vi "ProcessInfoGui.vi"() -> (1 "cancel":bool, 2 "PlateType":T1)   [LabVIEW 2016]
uses:
  Sequence/Sequence.PlateType.ctl
  InfoGui.Action.ctl
  tools/Translator/Translator.Message.ctl
  tools/Translator/Translator.FormatMessage.vi
  Sequence/Sequence.Global.vi
  Global/ApplicationGlobal.vi
  tools/Translator/Translator.Global.vi
panel:
  in  "CancelButton":bool
  in  "ClientPlateSelect":bool
  in  "WabcoPlateSelect":bool
  out "Message":string
  out "Client Plate Status":string caption="Status tabliczki Klienta"
  out "ClientPlate":picture
  out "Wabco Plate Status":string caption="Status tabliczki Wabco"
  out "WabcoPlate":picture
  out "_loop":i32(ring)=4
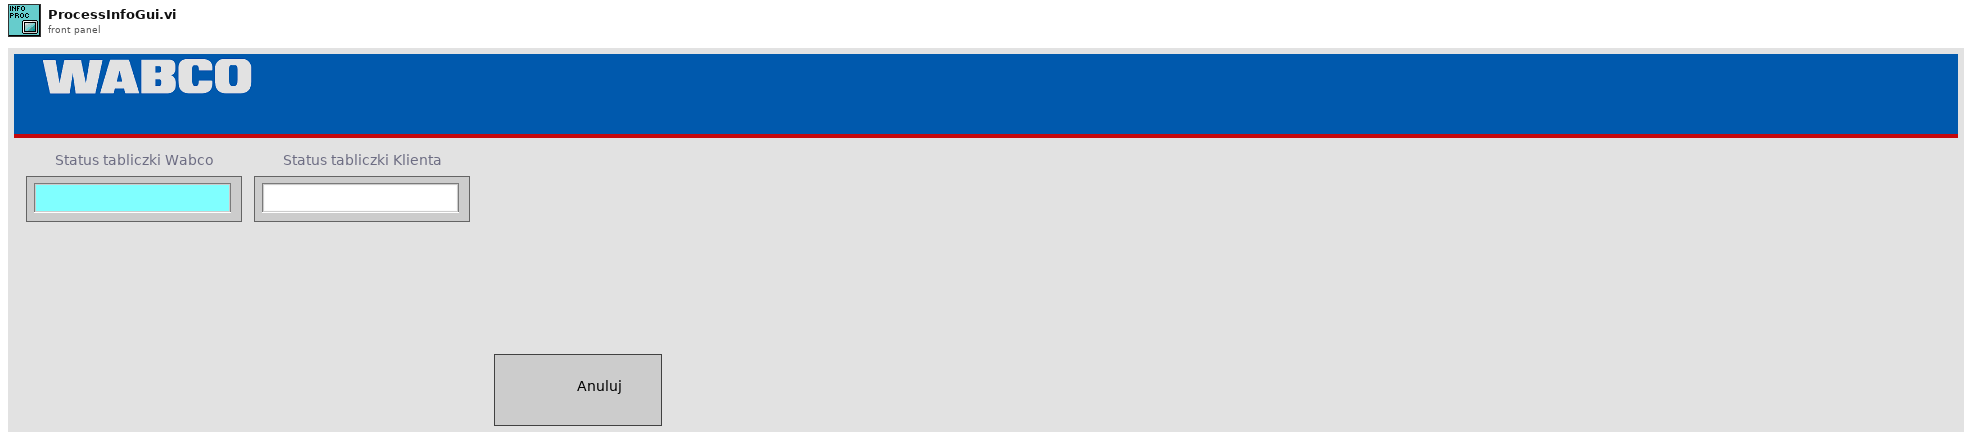
[diagram p1: front panel]
types:
  T1 = typedef "Sequence.PlateType.ctl" = enum16{"Wabco", "Client"}
  T2 = typedef "InfoGui.Action.ctl" = enum32{"idle", "constructor", "destructor", "--- InfoGUI ---"}
  T3 = typedef "Translator.Message.ctl" = enum16{"-", "Event confirmed", "Log out", "Log in", "Shutdown", "Cancel", "Start", "Begin time", "End time", "Duration", "Service Mode", "Ignore Results", "Serial Format", "On", "Off", "OK", "NOK", "NOK %s", "Home", "Work", "Close", "Open", "In progress...", "Missing", "Empty", "Hardware failure", "Initial", "Default", "Total", "Out of range", "Free disk space is below 1GB - contact technician", "Error %d >> %s", "Error %d >> %s >> %s", "Msg %d >> %s", "Laser msg %d %s", "Laser cmd error %s %d", "Laser cmd failed %s", "Laser cmd warning %s", "Laser disconnected", "Laser status %s", "Laser already started", "Laser job unkonwn %s", "Laser job missing %s", "Laser job select failure %s", "Unable to start laser printing (%s)", "Unable to stop laser printing (%s)", "Laser marking aborted", "Laser marking timeout", "Unable to reset Laser Interlock (%s)", "Unable to trigger Laser. Laser not ready (%s)", "Laser job '%s' coordinates not configured", "Starting %s", "Quitting %s", "Configured", "Initializing", "Quitting", "Loading", "Loaded %d results", "Loaded %d events", "Running", "Stopped", "Summary", "Laser", "Do you want to continue?", "Do you want to delete the configuration?", "The configuration is being used by an order. Unable to delete!", "Press confirm button", "Station is not based. Do you want to exit?", "Station requires changeover. Do you want to run the test?", "Test options are not set as default. Do you want to continue?", "Formatting of WabcoNo is disabled. Do you want to continue?", "Product not detected. Do you want to continue?", "Product scan failed. Do you want to continue?", "Calibration", "Log out?", "System", "All", "IDLE", "Translating...%s", "Not found", "Alarm %s", "Run", "Skip", "Abort", "Repeat", "Please wait...", "Database disconnected", "Database disconnected - changeover disabled!", "Login to database successful", "Login to database failed: %d; %s", "Unable to check the product status of reference %d - database disconnected", "Unable to set the product status of reference %d - database disconnected", "Variant file backup %s", "Read variant (%s)", "Result", "Station armed!", "Station requires changeover!", "Select reference number...", "EMERGENCY BUTTON - press Control button", "EMERGENCY DOOR - press Control button", "Resetting Emergency...", "Unable to reset safety circuit - Emergency Button pressed", "Unable to reset safety circuit - Emergency Side Door open", "Station not based", "Station based", "Station not empty", "Station basing...", "No order", "Press Start to begin new order", "Scanning new order", "Order NOK. Correct or scan again", "Order OK. Press Accept", "Order ready", "Revolver incorrect", "Fork incorrect", "Revolver missing", "Revolver empty", "Container missing", "Offline results", "Offline statistics", "Updating statistics %.1f %%", "DMC Configurator", "Door open", "Close the front door", "Press start button", "Done. Open the front door", "Running...", "Running...%.1f %%", "Pause %s", "Pause %s. NOK container missing", "Pause %s. OK container missing", "Pause %s. Revolver empty", "Pause %s. Revolver missing", "Pause %s. Revolver incorrect", "Pause %s. Fork missing", "Pause %s. Fork incorrect", "Pause %s. Too many failures", "Pause %s. Unloading failure", "Pause %s. One slot is not working", "Pause %s. Part order is done. Empty OK container", "Pause %s. Unable to move product to slot", "Pause %s. Unable to move back product pusher", "Pause %s. Unable to lift product", "Pause %s. Unable to move back product lifter", "Pause %s. Unable to move product arm to Work", "Pause %s. Unable to move product arm to NOK", "Pause %s. Unable to move product arm to OK", "Pause %s. Unable to unsuck the NOK product", "Pause %s. Unable to drop the NOK product", "Pause %s. Product OK missing", "Pause %s. Unable to unsuck the OK product", "Pause %s. Unable to drop the OK product", "Stopping...", "File '%s' is missing", "File '%s' is broken", "File '%s' is running", "Log file started (%s)", "Log file ended (%s)", "Log file stopped (%s)", "Log file ignored (%s)", "Log file exported (%s)", "Log file export failed (%s)", "Wrong serial number in log file", "Wrong reference number in log file", "Test steps are missing", "%s = %.3f", "Process param '%s' not found in DB", "Process param '%s' wrong order", "Process param '%s' value %.3f out of limits (%.3f; %.3f)", "Step%d param '%s' not found in DB", "Step%d param '%s' wrong order", "Step%d param '%s' value %.3f out of limits (%.3f; %.3f)", "Step%d EV '%s' not found in DB", "Step%d EV '%s' wrong order", "\"%s\" not found in DB", "\"%s\" wrong order", "\"%s\" value %.3f out of limits (%.3f; %.3f)", "\"%s\" not found in software", "Process init (%s)", "Process started", "Process restarted", "Process run", "Process done", "Process done - remove OK container", "Process aborted", "Process aborted at work", "Process aborted at home", "Process error", "Process error at home", "Process error at work", "Process close", "Process pause", "Process continue", "Process door open", "Process door close", "Process pause at slot %s due to %s", "Select plate from the order to process", "Do you want to start the process?", "Do you want to continue the process?", "There is unfinished order. Do you want to put the new order?", "Product %s %d OK", "Product %s %d NOK", "Unable to unload the slot %s. Product missing in the slot", "Unable to unload the slot %s. Product already in the arm", "Unable to accept the product as OK. Product missing in slot %s", "Unable to accept the product as OK. Product could not drop into the container at slot %s", "Unable to accept the product as NOK. Product could not drop into the container at slot %s", "Scan failed. Error %s", "Scan failed. Scanner disconnected", "Scan failed. Wrong Wabco number %d, limit (%d,%d)", "Scan failed. Wrong serial number %d, limit (%d,%d)", "Scan failed. Wrong date %d, limit (%d,%d)", "Scan failed. Wrong product wabco number %d (expected %d)", "Scan failed. Wrong product serial number %d (expected > 0)", "Scan OK %s", "Scan failed. Unable to determine table position (%s)", "Scan failed. Timeout", "Tune failed. Scanner disconnected", "Tune failed. Timeout", "%s = %d", "%s = %d->%d", "Unable to set %s = %.2f - Air Pressure Inside off", "Unable to set digital output '%s' = %d", "Unable to activate air pressure inside - timeout", "Unable to activate air pressure inside - aborted", "Unable to switch on Air Main Valve - Air Pressure Inlet off", "Unable to switch on Air Main Valve - Door open", "Unable to switch off Air Main Valve - timeout", "Unable to switch off Air Main Valve - aborted", "Unable to rotate Table - timeout", "Unable to rotate Table - aborted", "Unable to rotate Table - Product Move not in Home position", "Unable to rotate Table - Air Pressure Inside off", "Unable to rotate Table - Product Lift A not in Home position", "Unable to rotate Table - Product Lift B not in Home position", "Unable to rotate Table - unlock before movement timeout", "Unable to rotate Table - lock after movement timeout", "Unable to move Table Lock to %s position - timeout", "Unable to move Table Lock to %s position - aborted", "Unable to move Table Lock to %s position - Air Pressure Inside off", "Unable to move Table Lock to %s position - Table not in position", "Unable to move Product Lift A to %s position - timeout", "Unable to move Product Lift B to %s position - timeout", "Unable to move Product Lift A to %s position - aborted", "Unable to move Product Lift B to %s position - aborted", "Unable to move Product Lift A to %s position - Air Pressure Inside off", "Unable to move Product Lift B to %s position - Air Pressure Inside off", "Unable to move Product Lift A to %s position - Table not locked", "Unable to move Product Lift B to %s position - Table not locked", "Unable to move Product Lift A to %s position - Product Arm not in Work position", "Unable to move Product Lift B to %s position - Product Arm not in Work position", "Unable to set Product Suction Gripper %s to %s - timeout", "Unable to set Product Suction Gripper %s to %s - aborted", "Unable to set Product Suction Gripper %s to %s - Air Pressure Inside off", "Unable to set Product Suction Gripper %s to %s - Table slot unkown", "Unable to move Product Arm to %s position - timeout", "Unable to move Product Arm to %s position - aborted", "Unable to move Product Arm to %s position - Air Pressure Inside off", "Unable to move Product Arm to %s position - Product Lift A not in Home position", "Unable to move Product Arm to %s position - Product Lift B not in Home position", "Unable to move Product to %s position - timeout", "Unable to move Product to %s position - aborted", "Unable to move Product to %s position - Air Pressure Inside off", "Unable to move Product to %s position - Table not in position"}
  T4 = enum8{"Enabled", "Disabled", "Disabled and Grayed Out"}
  T5 = typedef "FestoCPX.Station.ButtonsState.ctl" = cluster{"Start":bool, "Stop":bool, "Control":bool}
  T6 = typedef "Sequence.Data.ctl" = cluster{"BeginTS":timestamp, "EndTS":timestamp, "State":T7, "Status.Work":T8, "Status.Process":T8, "Status.Home":T8, "Status.Wabco":T8, "Status.Client":T8, "BreakReason":T9, "BreakSource":T10, "DoorLock":bool, "Status.Prod":T11[], "UserAction":T15, "UserData":T16, "Error":errorcluster, "Code":T19, "Rotations":i32, "ProdIdx":i32, "ProdDone":T11[], "PrintedSerials-Wabco":i32[], "PrintedSerials-Client":i32[], "Counters-Wabco":T25, "Counters-Client":T25}
  T7 = typedef "Sequence.State.ctl" = enum16{"Init", "Idle", "Home", "Work", "Run", "Pause"}
  T8 = typedef "Sequence.Step.Status.ctl" = enum16{"-", "Pending", "Running", "Skipped", "Passed", "Failed", "Done", "Error", "Aborted", "Stopped"}
  T9 = typedef "Sequence.Test.BreakReason.ctl" = enum16{"-", "NOK container", "OK container", "Rev empty", "Rev missing", "Rev wrong", "Fork missing", "Fork wrong", "NOK limit", "Unload failure", "Single slot", "Part done", "Err: Prod move work", "Err: Prod move home", "Err: Prod lift work", "Err: Prod lift home", "Err: Prod Arm Work", "Err: Prod Arm NOK", "Err: Prod Arm OK", "Err: Prod NOK suck", "Err: Prod NOK drop", "Err: Prod OK missing", "Err: Prod OK suck", "Err: Prod OK drop"}
  T10 = typedef "Sequence.Test.BreakSource.ctl" = enum16{"-", "A", "B", "A/B"}
  T11 = typedef "Sequence.Test.Status.ctl" = cluster{"Slot":T12, "A":T14, "B":T14}
  T12 = typedef "Sequence.Slot.StatusData.ctl" = cluster{"ID":i32, "Unload":T13, "TS":timestamp, "duration":u32}
  T13 = typedef "Sequence.Test.Unload.Status.ctl" = enum16{"init", "check NOK", "check OK", "wait on NOK", "wait on OK", "wait on Unload", "done"}
  T14 = typedef "Sequence.Prod.StatusData.ctl" = cluster{"status":T8, "pause":T9, "present":bool, "printed":bool, "scanned":bool, "tuned":bool, "removed":bool, "OCRignored":bool, "LaserVariables":string[], "Serial":i32, "path":path, "corners":cluster{"X":i32, "Y":i32}[], "verification":u8, "ScanerReadOut":string[], "Caption":string}
  T15 = typedef "Sequence.UserActions.ctl" = cluster{"Stop":bool, "Pause":bool, "Next":bool}
  T16 = typedef "Sequence.UserData.ctl" = cluster{"GuiMode":T17, "Test":T18, "ContinueOrder":bool}
  T17 = typedef "Sequence.MainMode.ctl" = enum16{"Process", "Base", "Order", "Manual", "Logs", "Results", "Stats", "DMC Config"}
  T18 = typedef "MainGui.TestOptions.ctl" = cluster{"IgnoreResults":bool, "IgnoreImages":bool, "ServiceMode":bool, "IgnoreOCR":bool}
  T19 = typedef "Sequence.Code.Sets.ctl" = cluster{"Ready":bool, "DoubleOrder":bool, "OrderDone":bool, "AllowSingleSlot":bool, "IgnoreOCR":bool, "ThresholdA":u8, "ThresholdB":u8, "Plate":T1, "ImgPath":path, "Variant":T20}
  T20 = typedef "Logger.Variant.Sets.ctl" = cluster{"State":T21, "ImgPath":path, "WabcoPlate":string, "WabcoProduct":string, "ClientProduct":string, "ClientPlate":string, "TotalQuantity":u16, "OrderQuantity":u16, "Serial":i32, "Wabco":T22, "Client":T22}
  T21 = typedef "Station.Changeover.State.vi" = enum16{"Init", "Scaning", "NOK", "Wait for ack", "Ready"}
  T22 = typedef "Station.Plate.Properties.ctl" = cluster{"LaserJob":string, "AdditionalTxt":string, "FactoryCode":string, "RevID":u8, "ForkID":u8, "FailuresLimit":u16, "GlobalCnt":i32, "ScannerProgram":u8, "SerialFormat":T23, "CoordA":T24, "CoordB":T24, "DMCconfig":i32, "CVX_Program":u16}
  T23 = typedef "Sequence.Code.SerialFormat.ctl" = enum8{"", "6 dig", "7 dig"}
  T24 = typedef "V7310.Job.Sets.ctl" = cluster{"X":dbl, "Y":dbl, "Angle":dbl}
  T25 = typedef "Sequence.Counters.ctl" = cluster{"Expected":u16, "Done":u16, "OK":u16, "NOK":u16, "NOKlimit":u16, "Part":u16, "PartOK":u16}
  T26 = typedef "LVPositionTypeDef.ctl" = cluster{"Left":i32, "Top":i32}
  T27 = typedef "imagedata.ctl" = cluster{"image type":i32, "image depth":i32, "image":u8[], "mask":u8[], "colors":u32[], "Rectangle":cluster{"left":i16, "top":i16, "right":i16, "bottom":i16}}
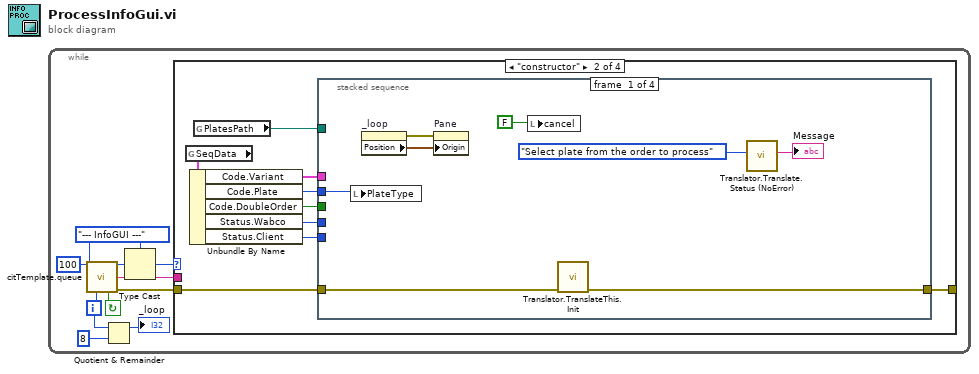
[diagram p0: block diagram]
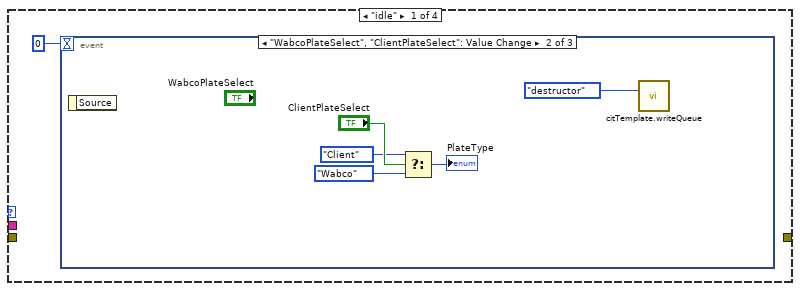
[diagram p2: hidden frame]
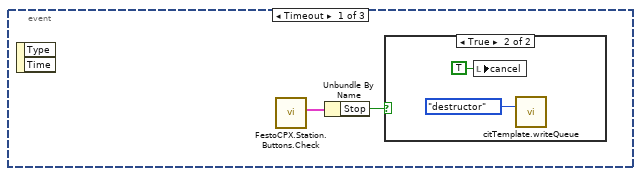
[diagram p3: hidden frame]
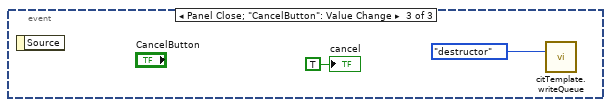
[diagram p5: hidden frame]
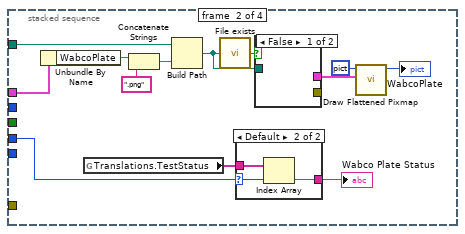
[diagram p6: hidden frame]
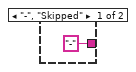
[diagram p7: hidden frame]
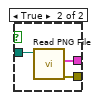
[diagram p8: hidden frame]
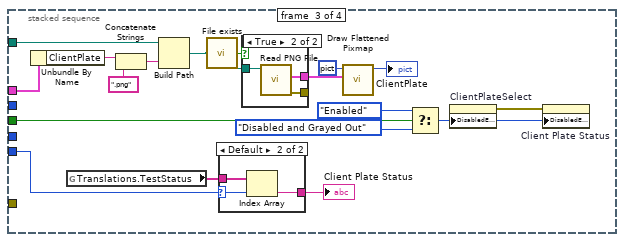
[diagram p9: hidden frame]
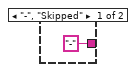
[diagram p10: hidden frame]
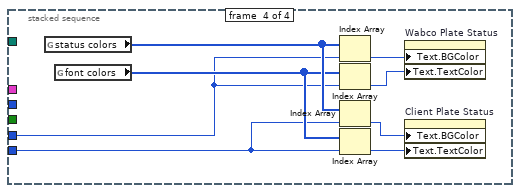
[diagram p12: hidden frame]
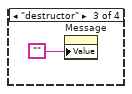
[diagram p13: hidden frame]
diagram:
  n1 = while {
    i -> [w1]
    stop <- w10 continue-if-true
    w4 = InfoGui.Action."--- InfoGUI ---" ("Action")
    n2 = call "citTemplate.queue.vi"("ms timeout (250 ms)"=100, "event enum"=w4, "iteration (-1)"=w1) -> ("event out"=w8:u32, "(flatten) data out"=w5:string, "continue"=w10:bool, "error out"=w6:errorcluster)  [unwired: 2 in, 7 out]
    n3 = Quotient & Remainder(x=w1, y=8) -> (x-y*floor(x/y)=→"_loop":i32)  [unwired: 1 out]
    n4 = Type Cast(type=w4, x=w8) -> (*(type *) &x=w7:T2)
    n5 = case shown="\"constructor\"" w7 {
      tunnel: w6 -> [_ w24 _ _]
      tunnel: w5 -> [_ _ _ _]
      tunnel: [_ w23 _ _] -> _
      frame "idle" {
        n6 = event shown="[1] \"WabcoPlateSelect\", \"ClientPlateSelect\": Value Change" {
          selector: _ -> [_ _ _]
          dyn-events: _ -> [_ _ _]
          timeout: 0 -> [_ _ _]
          event Timeout {
            n7 = event-data() -> ()  [unwired: 3 out]
            n8 = call "FestoCPX.Station.Buttons.Check.vi"() -> ("Buttons.State"=w13:T5)  [unwired: 10 in, 1 out]
            n9 = Unbundle By Name(w13) -> ("Stop"=w12:bool)
            n10 = case shown="True" w12 {
              frame False {
              }
              frame True {
                n11 = local write "cancel"(TRUE ("cancel")) -> ()
                n12 = call "citTemplate.writeQueue.vi"("event in (if not connected:all statemachine with data event)"=InfoGui.Action."destructor" ("Action")) -> ()  [unwired: 14 in, 1 out]
              }
            }
          }
          event "WabcoPlateSelect", "ClientPlateSelect": Value Change {
            n13 = event-data() -> ()  [unwired: 2 out]
            n14 = Select(t=Sequence.PlateType."Client" ("PlateType"), s="ClientPlateSelect", f=Sequence.PlateType."Wabco" ("PlateType")) -> (s? t:f=→"PlateType":T1)
            n15 = call "citTemplate.writeQueue.vi"("event in (if not connected:all statemachine with data event)"=InfoGui.Action."destructor" ("Action")) -> ()  [unwired: 14 in, 1 out]
          }
          event Panel Close; "CancelButton": Value Change {
            n16 = event-data() -> ()  [unwired: 2 out]
            n17 = call "citTemplate.writeQueue.vi"("event in (if not connected:all statemachine with data event)"=InfoGui.Action."destructor" ("Action")) -> ()  [unwired: 14 in, 1 out]
            "cancel" <- TRUE ("cancel")
          }
        }
      }
      frame "constructor" {
        n18 = global read "Sequence.Global.vi" "SeqData"() -> (w25:T6)
        n19 = Unbundle By Name(w25) -> ("Code.Variant"=w30:T20, "Code.Plate"=w29:T1, "Code.DoubleOrder"=w26:bool, "Status.Wabco"=w28:T8, "Status.Client"=w27:T8)
        n20 = global read "ApplicationGlobal.vi" "PlatesPath"() -> (w31:path)
        n21 = stacked-sequence {
          tunnel: w31 -> [_ w44 w70 _]
          tunnel: w30 -> [_ w40 w63 _]
          tunnel: w29 -> [w34 _ _ _]
          tunnel: w28 -> [_ w43 _ w90]
          tunnel: w27 -> [_ _ w62 w87]
          tunnel: w26 -> [_ _ w64 _]
          tunnel: w24 -> [w33 _ _ _]
          tunnel: [w32 _ _ _] -> w23
          frame #0 {
            n22 = local write "PlateType"(w34) -> ()
            n23 = property on="_loop" class="Ring (strict)"() -> (error out=w38:errorcluster, "Position"=w39:T26)  [unwired: 2 in, 1 out]
            n24 = property on="Pane" class="Pane"(error in=w38, "Origin"=w39) -> ()  [unwired: 1 in, 2 out]
            n25 = local write "cancel"(FALSE ("_b_ok")) -> ()
            n26 = call "Translator.TranslateThis.Init.vi"("error in"=w33) -> ("error out"=w32:errorcluster)  [unwired: 10 in]
            n27 = call "Translator.Translate.Status (NoError).vi"("msg"=Translator.Message."Select plate from the order to process" ("_Msg")) -> ("Translated Msg"=→"Message":string)  [unwired: 10 in]
          }
          frame #1 {
            n28 = Unbundle By Name(w40) -> ("WabcoPlate"=w49:string)
            n29 = global read "Translator.Global.vi" "Translations.TestStatus"() -> (w41:string[])
            n30 = Concatenate Strings(w49, ".png" ("string")) -> (w50:string)
            n31 = Build Path(base path=w44, name or relative path=w50) -> (appended path=w48:path)
            n32 = call "File exists.vi"("file path"=w48) -> ("exists?"=w47:bool)  [unwired: 4 in]
            n33 = case shown="Default" w43 {
              selector: w43 -> [_ w55]
              tunnel: ["-" ("String") w54] -> w42
              tunnel: w41 -> [_ w56]
              frame "-", "Skipped" {
              }
              frame Default {
                n34 = Index Array(array=w56, index=w55) -> (element=w54:string)
              }
            }
            "Wabco Plate Status" <- w42
            n35 = case shown="False" w47 {
              tunnel: w48 -> [_ w59]
              tunnel: [_ w58] -> w45
              tunnel: [_ w57] -> _
              frame False {
              }
              frame True {
                n36 = call <vilib>:"Read PNG File.vi"("path to PNG file"=w59) -> ("error out"=w57:errorcluster, "image data"=w58:T27)  [unwired: 8 in, 1 out]
              }
            }
            n37 = call <vilib>:"Draw Flattened Pixmap.vi"("image data"=w45, "picture"=picture data[5B]) -> ("new picture"=→"WabcoPlate":picture)  [unwired: 7 in]
          }
          frame #2 {
            n38 = Unbundle By Name(w63) -> ("ClientPlate"=w69:string)
            n39 = global read "Translator.Global.vi" "Translations.TestStatus"() -> (w61:string[])
            n40 = Concatenate Strings(w69, ".png" ("string")) -> (w75:string)
            n41 = Build Path(base path=w70, name or relative path=w75) -> (appended path=w74:path)
            n42 = call "File exists.vi"("file path"=w74) -> ("exists?"=w73:bool)  [unwired: 4 in]
            n43 = case shown="Default" w62 {
              selector: w62 -> [_ w80]
              tunnel: ["-" ("String") w79] -> w60
              tunnel: w61 -> [_ w81]
              frame "-", "Skipped" {
              }
              frame Default {
                n44 = Index Array(array=w81, index=w80) -> (element=w79:string)
              }
            }
            "Client Plate Status" <- w60
            n45 = case shown="True" w73 {
              tunnel: w74 -> [_ w84]
              tunnel: [_ w83] -> w71
              tunnel: [_ w82] -> _
              frame False {
              }
              frame True {
                n46 = call <vilib>:"Read PNG File.vi"("path to PNG file"=w84) -> ("error out"=w82:errorcluster, "image data"=w83:T27)  [unwired: 8 in, 1 out]
              }
            }
            n47 = call <vilib>:"Draw Flattened Pixmap.vi"("image data"=w71, "picture"=picture data[5B]) -> ("new picture"=→"ClientPlate":picture)  [unwired: 7 in]
            n48 = Select(t=T4."Enabled" ("Disabled"), s=w64, f=T4."Disabled and Grayed Out" ("Disabled")) -> (s? t:f=w66:T4)
            n49 = property on="ClientPlateSelect" class="Bool"("DisabledEnum"=w66) -> (error out=w65:errorcluster)  [unwired: 2 in, 1 out]
            n50 = property on="Client Plate Status" class="Str"(error in=w65, "DisabledEnum"=w66) -> ()  [unwired: 1 in, 2 out]
          }
          frame #3 {
            n51 = global read "ApplicationGlobal.vi" "status colors"() -> (w92:u32[])
            n52 = global read "ApplicationGlobal.vi" "font colors"() -> (w91:u32[])
            n53 = Index Array(array=w92, index=w90) -> (element=w89:u32)
            n54 = Index Array(array=w91, index=w90) -> (element=w88:u32)
            n55 = Index Array(array=w92, index=w87) -> (element=w86:u32)
            n56 = Index Array(array=w91, index=w87) -> (element=w85:u32)
            n57 = property on="Wabco Plate Status" class="Str"("Text.BGColor"=w89, "Text.TextColor"=w88) -> ()  [unwired: 2 in, 2 out]
            n58 = property on="Client Plate Status" class="Str"("Text.BGColor"=w86, "Text.TextColor"=w85) -> ()  [unwired: 2 in, 2 out]
          }
        }
      }
      frame "destructor" {
        n59 = property on="Message" class="Str"("Value"="") -> ()  [unwired: 2 in, 2 out]
      }
      frame "--- InfoGUI ---" {
      }
    }
  }
